vi "Set Core Count.vi"(8 "error in (no error)":errorcluster, 10 "Core Count":i32, 11 "CPU Info in":refnum<class "CPU Info.lvclass">) -> (0 "error out":errorcluster, 3 "CPU Info out":refnum<class "CPU Info.lvclass">)   [LabVIEW 2020, in "DSF Core.lvlib" / "CPU Info.lvclass"]
uses:
  CPU Info.lvclass
  CPU Info.lvclass/CPU Info.ctl
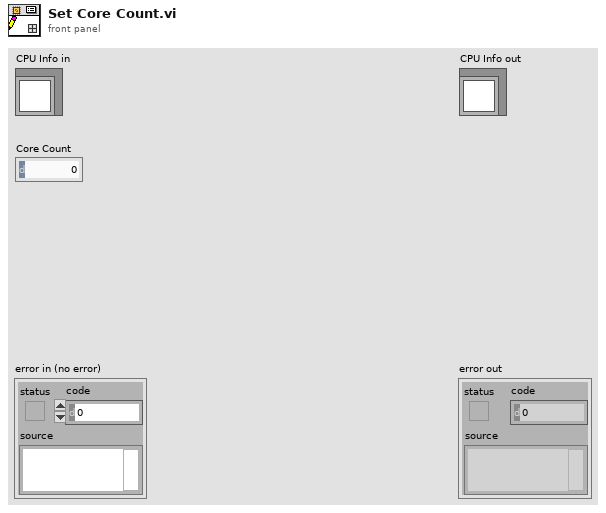
[diagram p1: front panel]
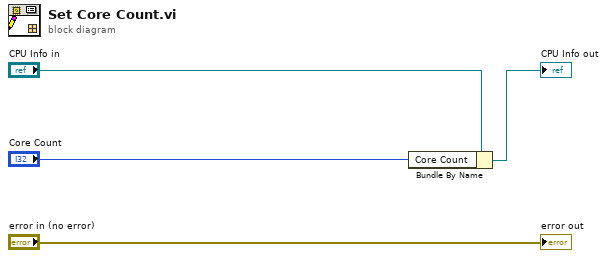
[diagram p0: block diagram]
diagram:
  n1 = Bundle By Name(cluster="CPU Info in", "Core Count"="Core Count") -> (→"CPU Info out":refnum<class "CPU Info.lvclass">)
  "error out" <- "error in (no error)"
